vi "Download Configuration File.vi"(8 "error in (no error)":errorcluster, 10 "Save config. as":path, 11 "VISA resource name":refnum<visa-resource-name>) -> (0 "error out":errorcluster, 3 "VISA resource name out":refnum<visa-resource-name>)   [LabVIEW 2017, in "Sefram DAS220.lvlib"]
doc: "Download the current device configuration in a file."
uses:
  <instrlib>/Sefram DAS220/Sefram DAS220.lvlib
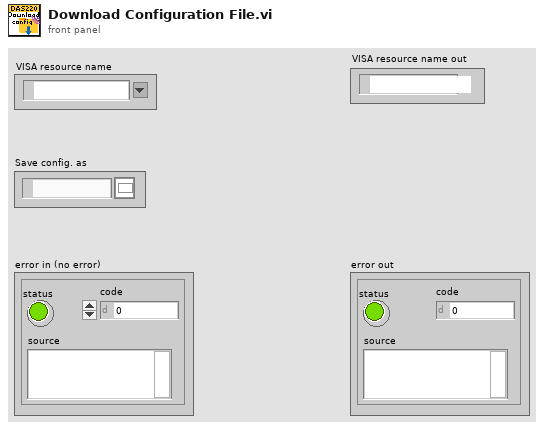
[diagram p1: front panel]
types:
  T1 = enum16{"open", "replace", "create", "open or create", "replace or create", "replace or create with confirmation"}
  T2 = enum16{"big-endian, network order", "native, host order", "little-endian"}
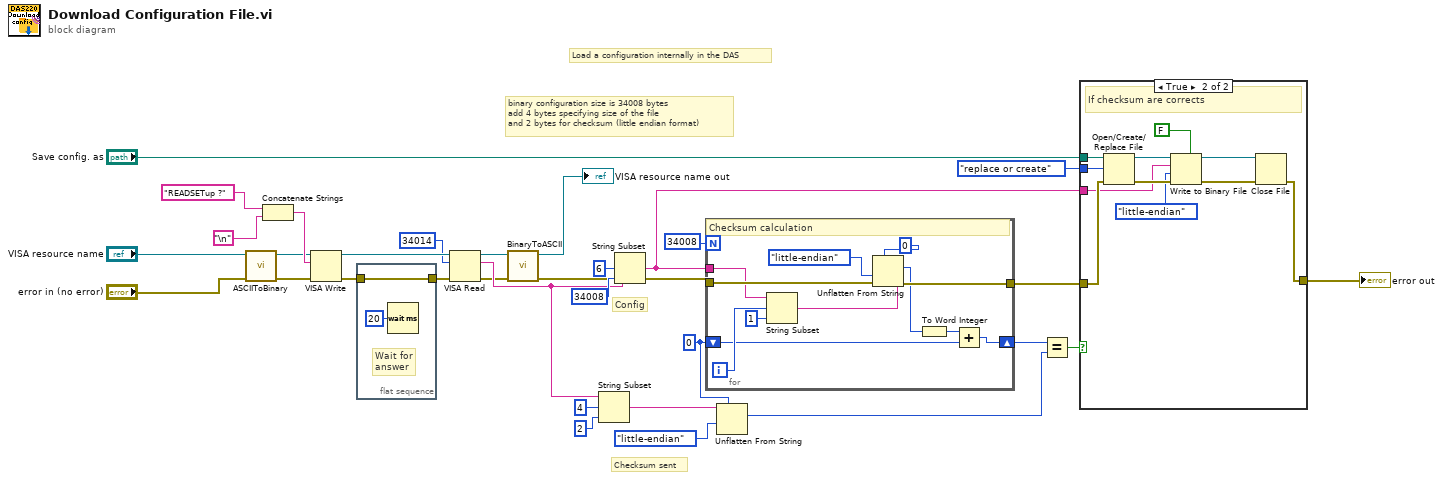
[diagram p0: block diagram]
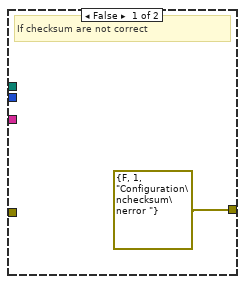
[diagram p2: hidden frame]
diagram:
  w17 = i16 0
  # "Checksum sent"
  # "Config"
  # "binary configuration size is 34008 bytes\nadd 4 bytes specifying size of the file \nand 2 bytes for checksum (little endian format)"
  # "Load a configuration internally in the DAS"
  n1 = call <instrlib>:"ASCIIToBinary.vi"("error in (no error)"="error in (no error)", "VISA resource name"="VISA resource name") -> ("error out"=w7:errorcluster, "VISA resource name"=w5:refnum<visa-resource-name>)  [unwired: 8 in]
  n2 = Concatenate Strings("READSETup ?" ("string"), "\n") -> (w32:string)
  n3 = VISA Write(VISA resource name=w5, write buffer=w32, error in (no error)=w7) -> (VISA resource name out=w29:refnum<visa-resource-name>, error out=w25:errorcluster)  [unwired: 1 out]
  n4 = flat-sequence {
    tunnel: w25 -> [w34]
    tunnel: [w34] -> w24
    frame #0 {
      # "Wait for\nanswer"
      n5 = Wait (ms)(milliseconds to wait=u32 20) -> ()  [unwired: 1 out]
    }
  }
  n6 = VISA Read(VISA resource name=w29, byte count=u32 34014, error in (no error)=w24) -> (VISA resource name out=w4:refnum<visa-resource-name>, read buffer=w18:string, error out=w3:errorcluster)  [unwired: 1 out]
  n7 = call <instrlib>:"BinaryToASCII.vi"("error in (no error)"=w3, "VISA resource name"=w4) -> ("error out"=w2:errorcluster, "VISA resource name"=→"VISA resource name out":refnum<visa-resource-name>)  [unwired: 8 in]
  n8 = String Subset(string=w18, offset (0)=4, length (rest)=2 ("length (rest)")) -> (substring=w21:string)
  n9 = String Subset(string=w18, offset (0)=6, length (rest)=34008 ("byte count")) -> (substring=w10:string)
  n10 = for {
    N: 34008 ("byte count") -> [_]
    tunnel: w2 -> [w46]
    tunnel: w10 -> [w45]
    tunnel: [w41] -> w11
    shift-right: [w38] -> w16
    shift-left: w17 -> [w39]
    i -> [w43]
    # "Checksum calculation"
    n11 = String Subset(string=w45, offset (0)=w43, length (rest)=1 ("length (rest)")) -> (substring=w40:string)
    n12 = Unflatten From String(type=u8 0, binary string=w40, byte order (0:big-endian, network order)=T2."little-endian", error in (no error)=w46) -> (value=w35:u8, error out=w41:errorcluster)  [unwired: 1 in, 1 out]
    n13 = To Word Integer(number=w35) -> (16bit integer=w36:i16)
    n14 = Add(x=w36, y=w39) -> (x+y=w38:i16)
  }
  n15 = Unflatten From String(type=w17, binary string=w21, byte order (0:big-endian, network order)=T2."little-endian") -> (value=w15:i16)  [unwired: 2 in, 2 out]
  n16 = Equal?(x=w16, y=w15) -> (x = y?=w14:bool)
  n17 = case shown="True" w14 {
    tunnel: T1."replace or create" ("operation (0:open)") -> [_ w58]
    tunnel: "Save config. as" -> [_ w57]
    tunnel: w11 -> [_ w56]
    tunnel: w10 -> [_ w51]
    tunnel: [errorcluster {"status"=FALSE, "code"=1, "source"="Configuration\nchecksum\nerror "} ("error constant") w48] -> w9
    frame False {
      # "If checksum are not correct"
    }
    frame True {
      # "If checksum are corrects"
      n18 = Open/Create/Replace File(file path (use dialog)=w57, error in=w56, operation (0:open)=w58) -> (refnum out=w55:refnum<file>, error out=w54:errorcluster)  [unwired: 3 in, 1 out]
      n19 = Write to Binary File(file (use dialog)=w55, data=w51, error in=w54, 5:FALSE ("prepend array or string size? (T)"), 9:T2."little-endian" ("byte order (0:big-endian, network order)")) -> (refnum out=w50:refnum<file>, error out=w49:errorcluster)  [unwired: 1 in, 1 out]
      n20 = Close File(refnum=w50, error in=w49) -> (error out=w48:errorcluster)  [unwired: 1 out]
    }
  }
  "error out" <- w9
